vi "Practica 02.vi"() -> ()   [LabVIEW 2011]
panel:
  in  "VISA COM IN":refnum<visa-resource-name>
  in  "stop":bool
  in  "Voltaje de salida":dbl(slide) scale=-10.0..10.0
  in  "SERVO ON":bool
  in  "INFO":bool
  # "Deslizador Lineal UTN"
  # "CONTOL DE VELOCIDAD"
  # "PRUEBAS BÁSICAS CON EL SERVOMOTOR"
  # "2. Especificar el voltaje de salida"
  # "1. Encender el servomotor"
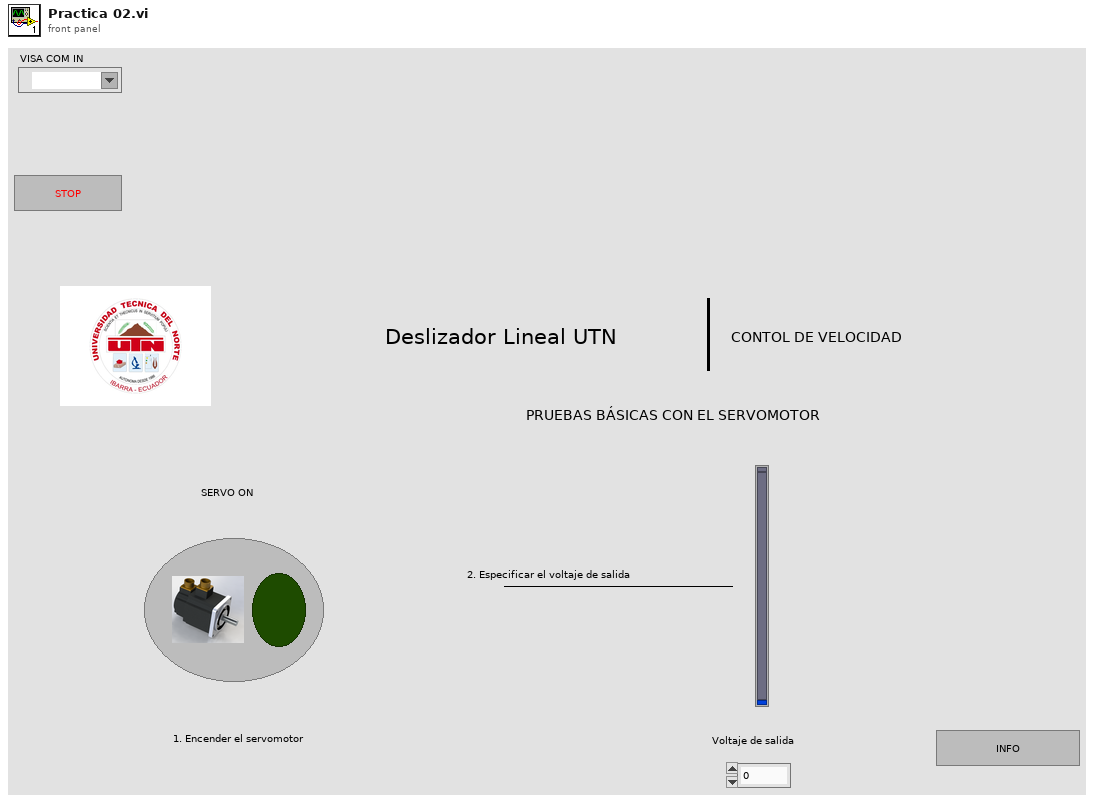
[diagram p1: front panel]
types:
  T1 = enum16{"Aout", "Fout", "Direccion", "ServoOn", "Idle"}
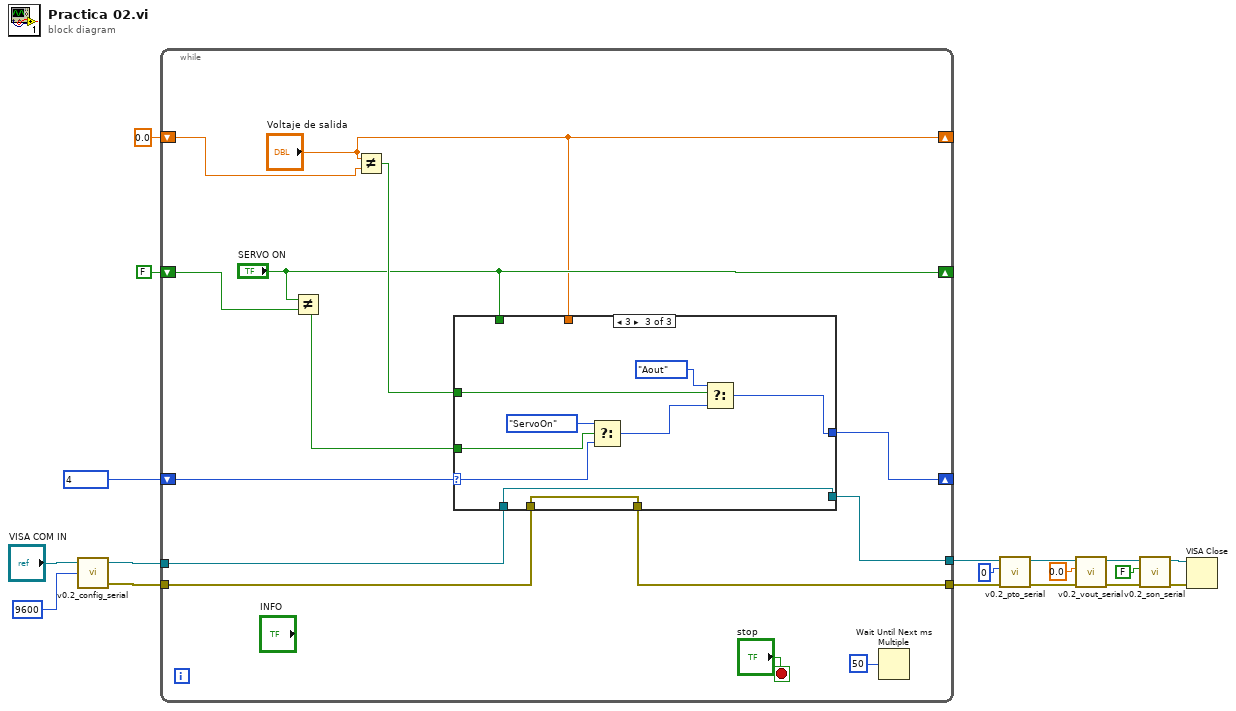
[diagram p0: block diagram]
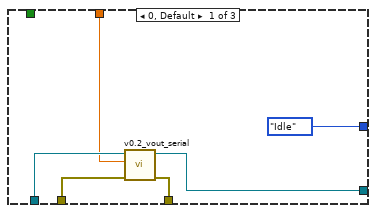
[diagram p2: hidden frame]
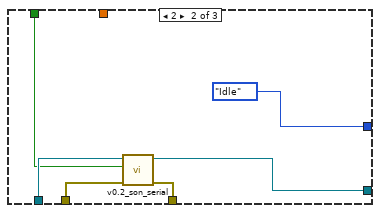
[diagram p3: hidden frame]
diagram:
  n1 = call "v0.2_config_serial.vi"("baud rate (9600/115200)"=u32 9600, "VISA COM IN"="VISA COM IN") -> ("error out"=w16:errorcluster, "VISA COM OUT"=w17:refnum<visa-resource-name>)  [unwired: 2 in]
  n2 = while {
    tunnel: w17 -> [w24]
    tunnel: w16 -> [w22]
    shift-right: ["Voltaje de salida"] -> _
    shift-left: 0.0 ("Volt") -> [w31]
    tunnel: [w21] -> w8
    shift-right: [w27] -> _
    shift-left: enum16{"Aout", "ServoOn", "Idle"} 4 -> [w29]
    shift-right: ["SERVO ON"] -> _
    shift-left: FALSE ("SON") -> [w26]
    tunnel: [w23] -> w12
    stop <- "stop" stop-if-true
    n3 = Not Equal?(x="SERVO ON", y=w26) -> (x != y?=w25:bool)
    n4 = Not Equal?(x="Voltaje de salida", y=w31) -> (x != y?=w28:bool)
    n5 = case shown="3" w29 {
      selector: w29 -> [_ _ w50]
      tunnel: w28 -> [_ _ w53]
      tunnel: [T1."Idle" T1."Idle" w45] -> w27
      tunnel: w25 -> [_ _ w49]
      tunnel: w24 -> [w38 w44 w48]
      tunnel: [w36 w42 w48] -> w23
      tunnel: "Voltaje de salida" -> [w37 _ _]
      tunnel: "SERVO ON" -> [_ w43 _]
      tunnel: w22 -> [w34 w40 w47]
      tunnel: [w33 w39 w47] -> w21
      frame 0, Default {
        n6 = call "v0.2_vout_serial.vi"("error in (no error)"=w34, "Volt"=w37, "VISA COM IN"=w38) -> ("error out"=w33:errorcluster, "VISA COM OUT"=w36:refnum<visa-resource-name>)  [unwired: 7 in]
      }
      frame 2 {
        n7 = call "v0.2_son_serial.vi"("error in (no error)"=w40, "ServoON"=w43, "VISA COM IN"=w44) -> ("error out"=w39:errorcluster, "VISA COM OUT"=w42:refnum<visa-resource-name>)  [unwired: 7 in]
      }
      frame 3 {
        n8 = Select(t=T1."ServoOn", s=w49, f=w50) -> (s? t:f=w46:u16)
        n9 = Select(t=T1."Aout", s=w53, f=w46) -> (s? t:f=w45:u16)
      }
    }
    n10 = Wait Until Next ms Multiple(millisecond multiple=u32 50) -> ()  [unwired: 1 out]
  }
  n11 = call "v0.2_pto_serial.vi"("error in (no error)"=w8, "Fout"=u32 0, "VISA COM IN"=w12) -> ("error out"=w7:errorcluster, "VISA COM OUT"=w11:refnum<visa-resource-name>)  [unwired: 7 in]
  n12 = call "v0.2_vout_serial.vi"("error in (no error)"=w7, "Volt"=0.0, "VISA COM IN"=w11) -> ("error out"=w6:errorcluster, "VISA COM OUT"=w10:refnum<visa-resource-name>)  [unwired: 7 in]
  n13 = call "v0.2_son_serial.vi"("error in (no error)"=w6, "ServoON"=FALSE, "VISA COM IN"=w10) -> ("error out"=w5:errorcluster, "VISA COM OUT"=w9:refnum<visa-resource-name>)  [unwired: 7 in]
  n14 = VISA Close(VISA resource name=w9, error in (no error)=w5) -> ()  [unwired: 1 out]
